vi "Global Buffer.vi"(7 "Clear":bool, 8 "Error In":errorcluster, 10 "Append":bool, 11 "Input String":string) -> (0 "Error Out":errorcluster, 3 "Output String":string)   [LabVIEW 2015]
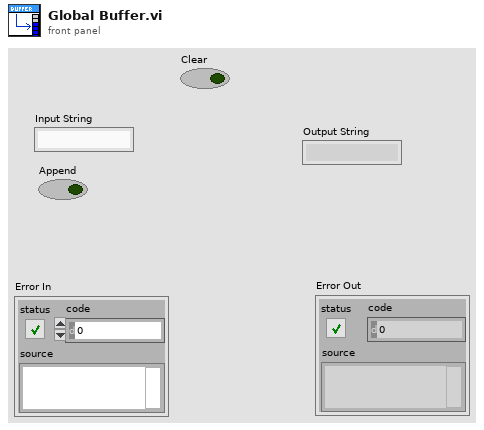
[diagram p1: front panel]
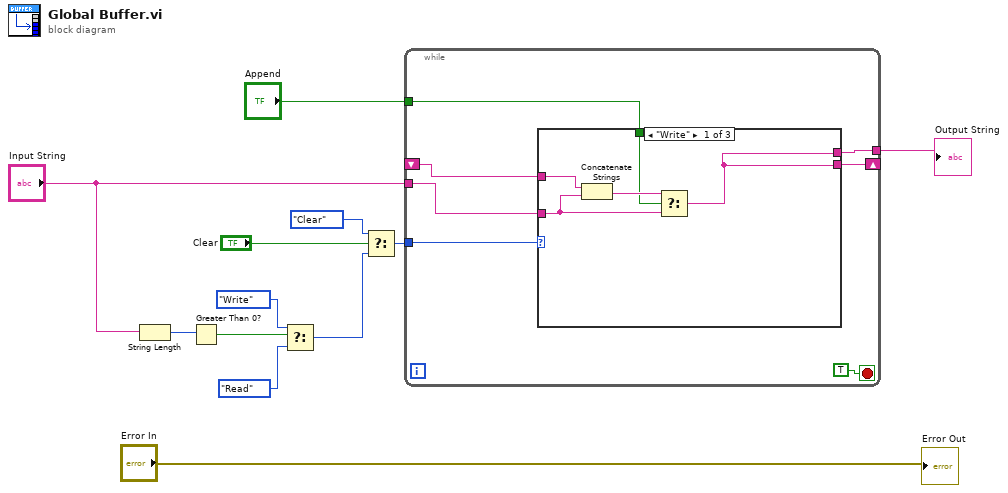
[diagram p0: block diagram]
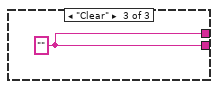
[diagram p3: hidden frame]
diagram:
  n1 = String Length(string="Input String") -> (length=w7:i32)
  n2 = Greater Than 0?(x=w7) -> (x > 0?=w6:bool)
  n3 = Select(t=enum16{"Write", "Read", "Clear"}."Write" ("Enum"), s=w6, f=enum16{"Write", "Read", "Clear"}."Read" ("Enum")) -> (s? t:f=w3:enum16{"Write", "Read", "Clear"})
  n4 = Select(t=enum16{"Write", "Read", "Clear"}."Clear" ("Enum"), s="Clear", f=w3) -> (s? t:f=w11:enum16{"Write", "Read", "Clear"})
  n5 = while {
    tunnel: "Input String" -> [w19]
    shift-right: [w18] -> _
    shift-left: _ -> [w16]
    tunnel: [w17] -> w9
    tunnel: w11 -> [w14]
    tunnel: "Append" -> [w13]
    stop <- TRUE stop-if-true
    n6 = case shown="\"Write\"" w14 {
      tunnel: w19 -> [w22 _ _]
      tunnel: [w21 w25 w26] -> w18
      tunnel: [w21 w25 w26] -> w17
      tunnel: w16 -> [w24 w25 _]
      tunnel: w13 -> [w20 _ _]
      frame "Write" {
        n7 = Concatenate Strings(w24, w22) -> (w23:string)
        n8 = Select(t=w23, s=w20, f=w22) -> (s? t:f=w21:string)
      }
      frame "Read", Default {
      }
      frame "Clear" {
        w26 = "" ("String")
      }
    }
  }
  "Output String" <- w9
  "Error Out" <- "Error In"
